vi "SetParam.vi"(8 "error in (no error)":errorcluster caption="entrée d'erreur (pas d'erreur)", 10 "contingency_matrix":cluster{"eps":string, "sparse":bool}={"eps"="None", "sparse"=FALSE}, 11 "Contingency_Matrix.lvclass":refnum<class "Contingency_Matrix.lvclass">) -> (0 "error out":errorcluster caption="sortie d'erreur", 3 "Contingency_Matrix.lvclass":refnum<class "Contingency_Matrix.lvclass">)   [LabVIEW 2020, in "Contingency_Matrix.lvclass"]
doc: "Set Parameters"
uses:
  Contingency_Matrix.lvclass
  Contingency_Matrix.lvclass/Contingency_Matrix.ctl
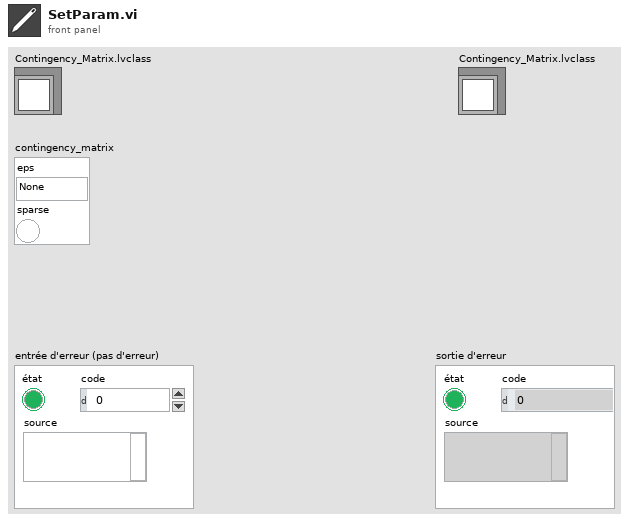
[diagram p1: front panel]
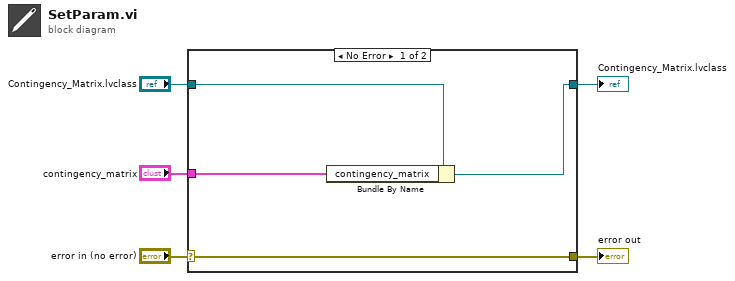
[diagram p0: block diagram]
diagram:
  n1 = case shown="No Error" "error in (no error)" {
    selector: "error in (no error)" -> [w9 w10]
    tunnel: [w9 w10] -> w4
    tunnel: [w7 w11] -> w2
    tunnel: "Contingency_Matrix.lvclass" -> [w8 w11]
    tunnel: "contingency_matrix" -> [w6 _]
    frame No Error {
      n2 = Bundle By Name(cluster=w8, "contingency_matrix"=w6) -> (w7:refnum<class "Contingency_Matrix.lvclass">)
    }
    frame Error {
    }
  }
  "error out" <- w4
  "Contingency_Matrix.lvclass" <- w2
